vi "LimeSDR_TwoTone_Tx_LabVIEW_V1.0.vi"() -> ()   [LabVIEW 2018, in "LMS_LV_Drv.lvlib"]
uses:
  LMS_LV_Drv.lvlib
  Stream_ctl.ctl
panel:
  in  "stream_In":T1={"handle"=0, "isTx"=1, "channel"=0, "fifoSize"=1000000, "throughputVsLatency"=0.5, "dataFmt"=0}
  out "return":i32=2098176
  in  "Direction":u8(ring) items=["RX", "TX"]
  out "EXIT":bool=TRUE
  in  "stop":bool
  in  "FM  Frequency":dbl(slide)=500000000.0 min=85000000.0 max=108000000.0 step=50000.0 scale=85000000.0..108000000.0 scale format="%#_6p"
  in  "chan":u64
  out "LimeSDR_info":string="LimeSDR-USB, media=USB 3.0, module=FX3, serial=0009072C02891115, index=0"
  in  "Sample Rate":dbl=20000000.0 format="%#_6p"
  out "error out":errorcluster
  # "Two Tone Generation Demo"
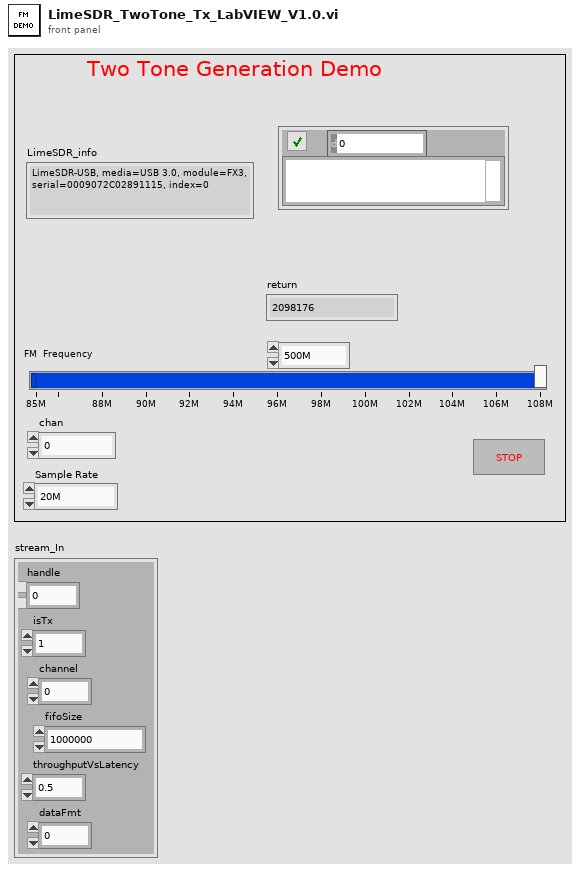
[diagram p1: front panel]
types:
  T1 = typedef "Stream_ctl.ctl" = cluster{"handle":u64, "isTx":u8, "channel":u32, "fifoSize":u32, "throughputVsLatency":dbl, "dataFmt":u32}
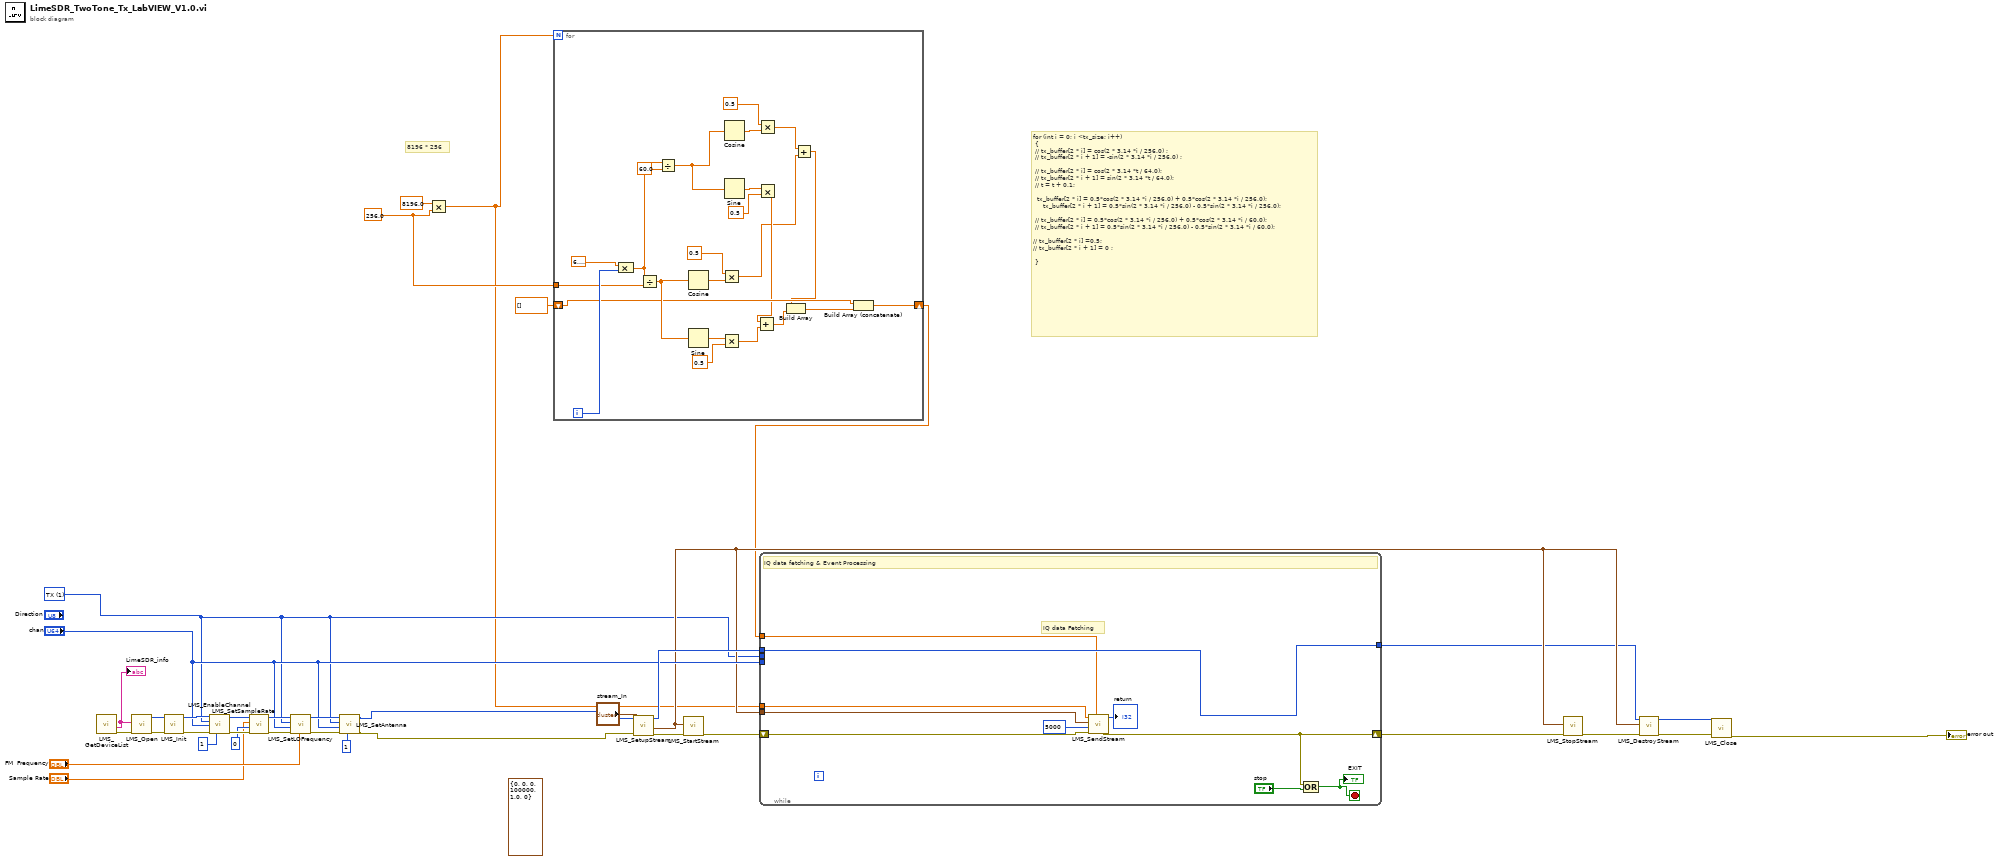
[diagram p0: block diagram]
diagram:
  w6 = 256.0 ("x")
  w11 = u8 1 items=["RX", "TX"] ("Direction")
  (unwired) T1 {"handle"=0, "isTx"=0, "channel"=0, "fifoSize"=100000, "throughputVsLatency"=1.0, "dataFmt"=0} ("stream")
  # "8196 * 256"
  # "for (int i = 0; i <tx_size; i++)\n\t{\n\t//\ttx_buffer[2 * i] = cos(2 * 3.14 *i / 256.0) ;\n\t//\ttx_buffer[2 * i + 1] = -sin(2 * 3.14 *i / 256.0) ;\n\n\t//\ttx_buffer[2 * i] = cos(2 * 3.14 *t / 64.0);\n\t//\ttx_buffer[2 * i + 1] = sin(2 * 3.14 *t / 64.0);\n\t//\tt = t + 0.1;\n\n\t\ttx_buffer[2 * i] = 0.5*cos(2 * 3.14 *i / 256.0) + 0.5*cos(2 * 3.14 *i / 256.0);\n    \ttx_buffer[2 * i + 1] = 0.5*sin(2 * 3.14 *i / 256.0) - 0.5*sin(2 * 3.14 *i / 256.0);\n\n\t//\ttx_buffer[2 * i] = 0.5*cos(2 * 3.14 *i / 256.0) + 0.5*cos(2 * 3.14 *i / 60.0);\n\t//\ttx_buffer[2 * i + 1] = 0.5*sin(2 * 3.14 *i / 256.0) - 0.5*sin(2 * 3.14 *i / 60.0);\n\n//\ttx_buffer[2 * i] =0.5;\n//\ttx_buffer[2 * i + 1] = 0 ;\n\n\t}"
  n1 = call "LMS_GetDeviceList.vi"() -> ("error out"=w37:errorcluster, "lms_info_str_t"=w36:string)  [unwired: 9 in, 1 out]
  "LimeSDR_info" <- w36
  n2 = call "LMS_Open.vi"("error in (no error)"=w37, "lms_info_str_t"=w36) -> ("error out"=w35:errorcluster, "device"=w34:i64)  [unwired: 8 in]
  n3 = call "LMS_Init.vi"("error in (no error)"=w35, "device_In"=w34) -> ("error out"=w27:errorcluster, "device_Out"=w28:i64)  [unwired: 8 in]
  n4 = call "LMS_EnableChannel.vi"("device_In"=w28, "dir_tx"=w11, "chan"="chan", "error in (no error)"=w27, "enabled"=i8 1) -> ("device_Out"=w24:i64, "error out"=w25:errorcluster)  [unwired: 9 in]
  n5 = call "LMS_SetSampleRate.vi"("error in (no error)"=w25, "oversample"=u64 0, "rate"="Sample Rate", "device_In"=w24) -> ("error out"=w23:errorcluster, "device_Out"=w22:i64)  [unwired: 6 in]
  n6 = call "LMS_SetLOFrequency.vi"("frequency"="FM  Frequency", "error in (no error)"=w23, "chan"="chan", "dir_tx"=w11, "device_In"=w22) -> ("error out"=w20:errorcluster, "device_Out"=w19:i64)  [unwired: 5 in]
  n7 = call "LMS_SetAntenna.vi"("index"=u64 1, "error in (no error)"=w20, "chan"="chan", "dir_tx"=w11, "device_In"=w19) -> ("error out"=w8:errorcluster, "device_Out"=w9:i64)  [unwired: 5 in]
  n8 = Multiply(x=8196.0, y=w6) -> (x*y=w3:dbl)
  n9 = for {
    N: w3 -> [_]
    tunnel: w6 -> [w59]
    shift-right: [w52] -> w4
    shift-left: dbl[] [] -> [w51]
    i -> [w60]
    n10 = Compound Arithmetic op=MULTIPLY(6.283185307179586, w60) -> (w50:dbl)
    n11 = Divide(x=w50, y=w59) -> (x/y=w56:dbl)
    n12 = Divide(x=w50, y=60.0) -> (x/y=w44:dbl)
    n13 = Cosine(x=w56) -> (cos(x)=w58:dbl)
    n14 = Sine(x=w56) -> (sin(x)=w55:dbl)
    n15 = Multiply(x=0.5, y=w58) -> (x*y=w41:dbl)
    n16 = Multiply(x=w55, y=0.5 ("x")) -> (x*y=w40:dbl)
    n17 = Cosine(x=w44) -> (cos(x)=w45:dbl)
    n18 = Sine(x=w44) -> (sin(x)=w47:dbl)
    n19 = Multiply(x=0.5, y=w45) -> (x*y=w43:dbl)
    n20 = Multiply(x=w47, y=0.5 ("x")) -> (x*y=w42:dbl)
    n21 = Add(x=w42, y=w40) -> (x+y=w38:dbl)
    n22 = Add(x=w43, y=w41) -> (x+y=w39:dbl)
    n23 = Build Array(w39, w38) -> (w53:dbl[])
    n24 = Build Array (concatenate)(w51, w53) -> (w52:dbl[])
  }
  n25 = call "LMS_SetupStream.vi"("error in (no error)"=w8, "stream_In"="stream_In", "device_In"=w9) -> ("error out"=w33:errorcluster, "steam_Out"=w13:T1, "device_Out"=w15:i64)  [unwired: 6 in]
  n26 = call "LMS_StartStream.vi"("error in (no error)"=w33, "stream 2"=w13) -> ("error out"=w16:errorcluster)  [unwired: 9 in]
  n27 = while {
    tunnel: w13 -> [w67]
    shift-right: [w66] -> w29
    shift-left: w16 -> [w68]
    tunnel: w15 -> [w71]
    tunnel: w11 -> [_]
    tunnel: "chan" -> [_]
    tunnel: [w71] -> w12
    tunnel: w4 -> [w65]
    tunnel: w3 -> [w64]
    stop <- w70 stop-if-true
    # "IQ data Fetching"
    # "IQ data fetching & Event Processing"
    n28 = call "LMS_SendStream.vi"("samples"=w65, "error in (no error)"=w68, "timeout_ms"=u64 5000, "stream"=w67, "sample_count"=w64) -> ("error out"=w66:errorcluster, "return"=→"return":i32)  [unwired: 5 in]
    n29 = Compound Arithmetic op=OR(w66, "stop") -> (w70:bool)
    "EXIT" <- w70
  }
  n30 = call "LMS_StopStream.vi"("error in (no error)"=w29, "stream"=w13) -> ("error out"=w30:errorcluster)  [unwired: 9 in]
  n31 = call "LMS_DestroyStream.vi"("error in (no error)"=w30, "stream"=w13, "device_In"=w12) -> ("error out"=w32:errorcluster, "device_Out"=w31:i64)  [unwired: 7 in]
  n32 = call "LMS_Close.vi"("error in (no error)"=w32, "device_In"=w31) -> ("error out"=→"error out":errorcluster)  [unwired: 9 in]
